vi "Dialog Box - Numeric Input.vi"(7 "Timeout (Seconds)":i16=-1, 8 "error in (no error)":errorcluster, 9 "Value In":dbl, 11 "Text":string) -> (0 "error out":errorcluster, 1 "Value Out":dbl)   [LabVIEW 2011]
doc: "Displays a simple one button dialog box with a numeric entry field.\n\nA timeout can be set. If no timeout is defined then the dialog will wait forever.\n\nThis dialog box will increase in size if required depending on the supplied text."
uses:
  <vilib>/Utility/miscctls.llb/LVSelectionTypeDef.ctl
panel:
  in  "OK Button":bool
  out "String":string
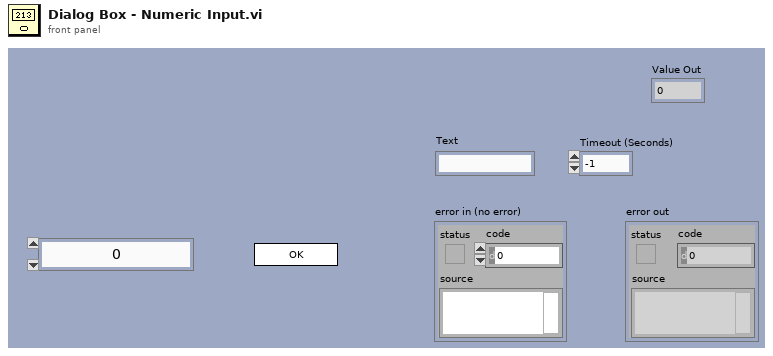
[diagram p1: front panel]
types:
  T1 = enum32{"Invalid", "Default", "Floating", "Floating/Auto-Hide", "Modal"}
  T2 = typedef "LVSelectionTypeDef.ctl" = cluster{"Selection Start":u32, "Selection End":u32}
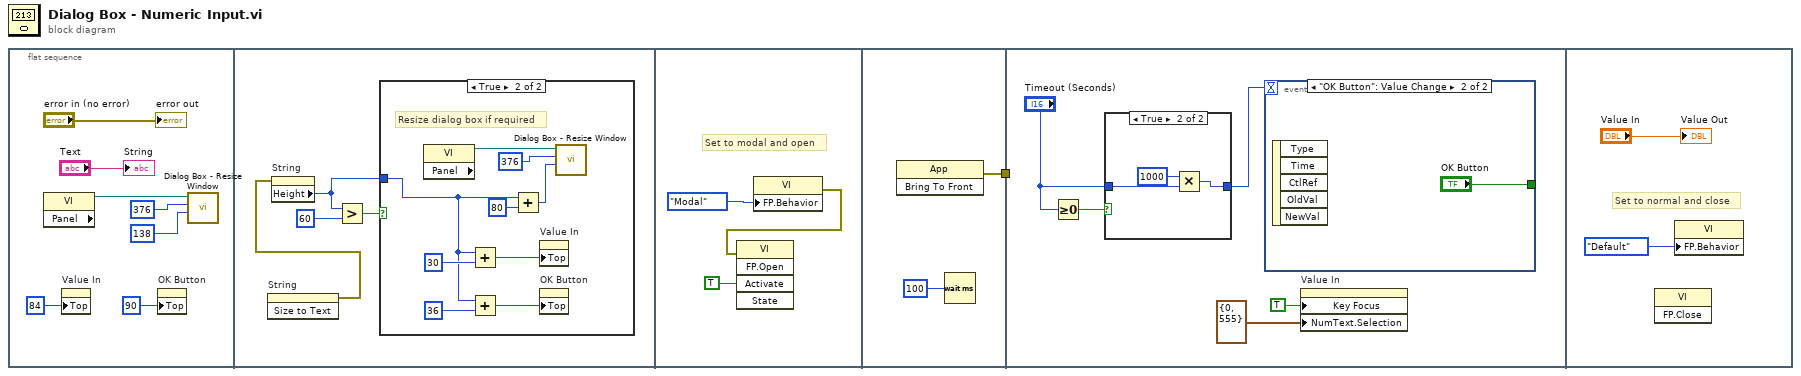
[diagram p0: block diagram]
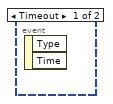
[diagram p3: hidden frame]
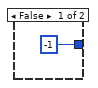
[diagram p4: hidden frame]
diagram:
  n1 = flat-sequence {
    tunnel: [w26] -> w1
    tunnel: w1 -> [_]
    frame #0 {
      n2 = property class="VI" props=["Panel"]() -> (reference out=w6:refnum<vi>)  [unwired: 2 in, 2 out]
      n3 = property on="Value In" class="DigNum (strict)"("Top"=84 ("Position:Top")) -> ()  [unwired: 2 in, 2 out]
      n4 = property on="OK Button" class="Bool"("Top"=90 ("Position:Top")) -> ()  [unwired: 2 in, 2 out]
      n5 = call "Dialog Box - Resize Window.vi"("Height"=i16 138, "Width"=i16 376, "reference"=w6) -> ()  [unwired: 8 in, 1 out]
      "String" <- "Text"
      "error out" <- "error in (no error)"
    }
    frame #1 {
      n6 = invoke on="String" class="Str" method="Size to Text"() -> (error out=w9:errorcluster)  [unwired: 3 in, 2 out]
      n7 = property on="String" class="Str"(error in=w9) -> ("Height"=w10:u32)  [unwired: 1 in, 2 out]
      n8 = Greater?(x=w10, y=u32 60) -> (0:w11:bool)
      n9 = case shown="True" w11 {
        tunnel: w10 -> [_ w14]
        frame False {
        }
        frame True {
          # "Resize dialog box if required"
          n10 = property class="VI" props=["Panel"]() -> (reference out=w21:refnum<vi>)  [unwired: 2 in, 2 out]
          n11 = Add(x=w14, y=u32 30) -> (x+y=w16:u32)
          n12 = Add(x=w14, y=u32 36) -> (x+y=w15:u32)
          n13 = Add(x=w14, y=u32 80) -> (x+y=w19:u32)
          n14 = property on="Value In" class="DigNum (strict)"("Top"=w16) -> ()  [unwired: 2 in, 2 out]
          n15 = property on="OK Button" class="Bool"("Top"=w15) -> ()  [unwired: 2 in, 2 out]
          n16 = call "Dialog Box - Resize Window.vi"("Height"=w19, "Width"=i16 376, "reference"=w21) -> ()  [unwired: 8 in, 1 out]
        }
      }
    }
    frame #2 {
      # "Set to modal and open"
      n17 = property class="VI"("FP.Behavior"=T1."Modal" ("Front Panel Window:Behavior")) -> (error out=w22:errorcluster)  [unwired: 2 in, 1 out]
      n18 = invoke class="VI" method="FP.Open"(error in=w22, "Activate"=TRUE ("Activate?")) -> ()  [unwired: 3 in, 5 out]
    }
    frame #3 {
      n19 = invoke class="App" method="Bring To Front"() -> (error out=w26:errorcluster)  [unwired: 3 in, 2 out]
      n20 = Wait (ms)(milliseconds to wait=u32 100) -> ()  [unwired: 1 out]
    }
    frame #4 {
      n21 = Greater Or Equal To 0?(x="Timeout (Seconds)") -> (x >= 0?=w31:bool)
      n22 = case shown="True" w31 {
        tunnel: "Timeout (Seconds)" -> [_ w36]
        tunnel: [i16 -1 w34] -> w29
        frame False {
        }
        frame True {
          n23 = Multiply(x=i16 1000, y=w36) -> (x*y=w34:i16)
        }
      }
      n24 = event shown="[1] \"OK Button\": Value Change" {
        selector: _ -> [_ _]
        dyn-events: _ -> [_ _]
        timeout: w29 -> [_ _]
        tunnel: [_ "OK Button"] -> _
        event Timeout {
          n25 = event-data() -> ()  [unwired: 1 in, 2 out]
        }
        event "OK Button": Value Change {
          n26 = event-data() -> ()  [unwired: 1 in, 5 out]
        }
      }
      n27 = property on="Value In" class="DigNum (strict)"("Key Focus"=TRUE, "NumText.Selection"=T2 {"Selection Start"=0, "Selection End"=555} ("Numeric Text.Selection")) -> ()  [unwired: 2 in, 2 out]
    }
    frame #5 {
      # "Set to normal and close"
      n28 = invoke class="VI" method="FP.Close"() -> ()  [unwired: 3 in, 3 out]
      n29 = property class="VI"("FP.Behavior"=T1."Default" ("Front Panel Window:Behavior")) -> ()  [unwired: 2 in, 2 out]
      "Value Out" <- "Value In"
    }
  }
